vi "UnpackASCIIString.vi"(8 "Error In":errorcluster, 11 "Packed\nByte Array":u8[](array[numeric])=[52, 96, 237, 199, 44, 244] format="%x") -> (0 "Error Out":errorcluster, 3 "string":string="MFC-1234")   [LabVIEW 2016, in "Brooks MFC.lvclass"]
doc: "Reconstruction of ASCII characters from Packed (6bist ASCII) data format"
uses:
  Brooks MFC.lvclass
panel:
  out "Boolean 2D array":bool[][](array[boolean])
  # "Example: \n(Hex) 34 60 ED   C7 2C F4\ntransforms to \"MFC-1234\""
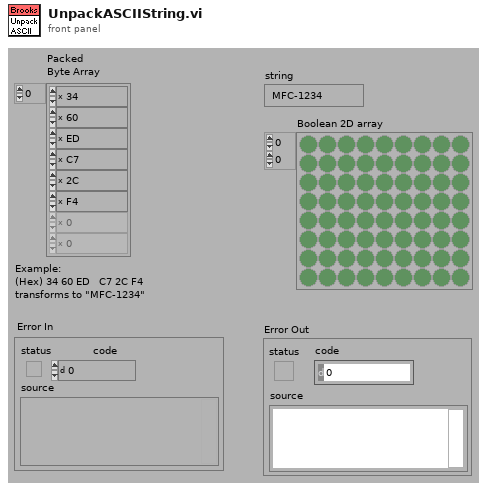
[diagram p1: front panel]
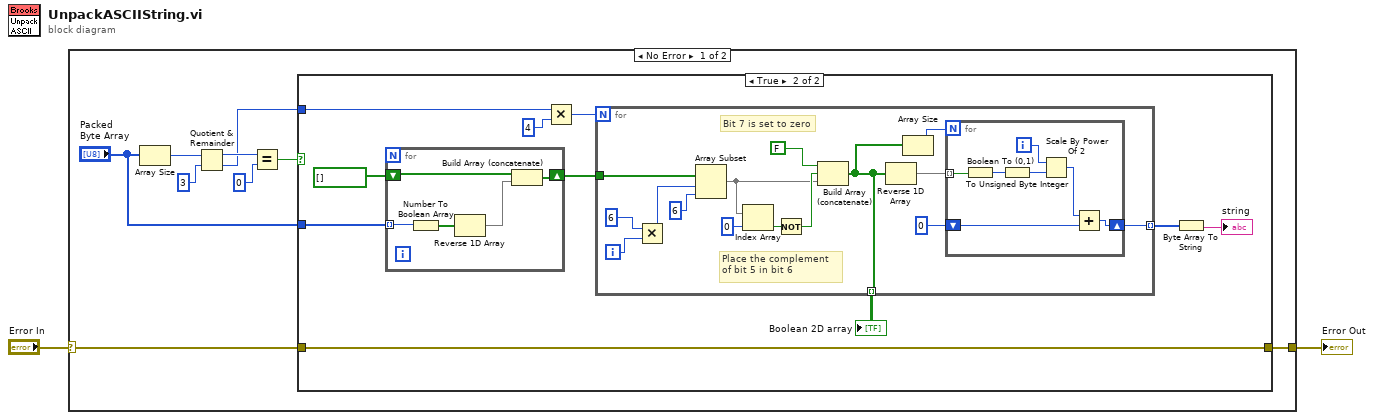
[diagram p0: block diagram]
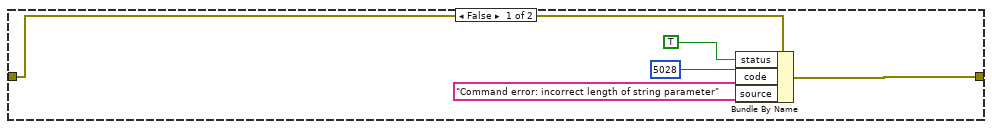
[diagram p2: hidden frame]
diagram:
  n1 = case shown="No Error" "Error In" {
    selector: "Error In" -> [w3 w54]
    tunnel: [w4 w54] -> w2
    frame No Error {
      n2 = Array Size(array="Packed\nByte Array") -> (size(s)=w11:i32)
      n3 = Quotient & Remainder(x=w11, y=3) -> (x-y*floor(x/y)=w9:i32, floor(x/y)=w5:i32)
      n4 = Equal?(x=w9, y=0) -> (x = y?=w7:bool)
      n5 = case shown="True" w7 {
        tunnel: "Packed\nByte Array" -> [_ w25]
        tunnel: w5 -> [_ w23]
        tunnel: [w15 w17] -> w4
        tunnel: w3 -> [w16 w17]
        frame False {
          n6 = Bundle By Name(cluster=w16, "status"=TRUE, "code"=5028, "source"="Command error: incorrect length of string parameter") -> (w15:errorcluster)
        }
        frame True {
          n7 = for {
            tunnel: w25 -> [w53] mode=indexing
            shift-right: [w51] -> w21
            shift-left: bool[] [] ("Boolean array 2") -> [w52]
            n8 = Number To Boolean Array(number=w53) -> (Boolean array=w50:bool[])
            n9 = Reverse 1D Array(array=w50) -> (reversed array=w49:bool[])
            n10 = Build Array (concatenate)(w52, w49) -> (w51:bool[])
          }
          n11 = Multiply(x=w23, y=i16 4) -> (x*y=w22:i32)
          n12 = for {
            N: w22 -> [_]
            tunnel: w21 -> [w41]
            tunnel: [w34] -> w20 mode=indexing
            tunnel: [w27] -> w18 mode=indexing
            i -> [w39]
            # "Bit 7 is set to zero"
            # "Place the complement\nof bit 5 in bit 6"
            n13 = Multiply(x=6, y=w39) -> (x*y=w37:i32)
            n14 = Array Subset(array=w41, index=w37, length=6) -> (w29:bool[])
            n15 = Index Array(array=w29, index=0) -> (element=w31:bool)
            n16 = Not(x=w31) -> (.not. x?=w30:bool)
            n17 = Build Array (concatenate)(FALSE, w30, w29) -> (w27:bool[])
            n18 = Reverse 1D Array(array=w27) -> (reversed array=w28:bool[])
            n19 = Array Size(array=w27) -> (size(s)=w35:i32)
            n20 = for {
              N: w35 -> [_]
              shift-right: [w45] -> w34
              shift-left: u8 0 -> [w46]
              tunnel: w28 -> [w42] mode=indexing
              i -> [w43]
              n21 = Boolean To (0,1)(Boolean=w42) -> (0, 1=w48:i16)
              n22 = To Unsigned Byte Integer(number=w48) -> (unsigned 8bit integer=w44:u8)
              n23 = Scale By Power Of 2(n=w43, x=w44) -> (x*2^n=w47:u8)
              n24 = Add(x=w47, y=w46) -> (x+y=w45:u8)
            }
          }
          "Boolean 2D array" <- w18
          n25 = Byte Array To String(unsigned byte array=w20) -> (string=→"string":string)
        }
      }
    }
    frame Error {
    }
  }
  "Error Out" <- w2
